vi "Calculate No of Scripts.vi"(0 "Sizes of Arrays":i32[](array[numeric]), 5 "Linked? Array":bool[](array[boolean])) -> (4 "No of scripts":i32)   [LabVIEW 2020, in "TALOS.lvlib" / "Run Utilities.lvlib" / "Scan SBlock.lvclass"]
doc: "Creates an array of parameter's values on range <From> to <To> with either step size or number of steps. It also returns a size of the array."
uses:
  Scan SBlock.lvclass
  Scan SBlock.lvclass/Scan SBlock.ctl
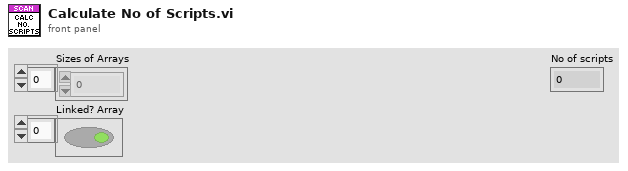
[diagram p1: front panel]
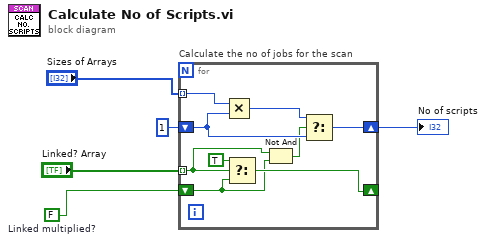
[diagram p0: block diagram]
diagram:
  w2 = FALSE  # Linked multiplied?
  n1 = for "Calculate the no of jobs for the scan" {
    tunnel: "Sizes of Arrays" -> [w14] mode=indexing
    shift-right: [w12] -> w1
    shift-left: 1 -> [w7]
    tunnel: "Linked? Array" -> [w9] mode=indexing
    shift-right: [w11] -> _
    shift-left: w2 -> [w10]
    n2 = Multiply(x=w14, y=w7) -> (x*y=w8:i32)
    n3 = Select(t=TRUE, s=w9, f=w10) -> (s? t:f=w11:bool)
    n4 = Not And(1:w10, 2:w9) -> (0:w6:bool)
    n5 = Select(t=w8, s=w6, f=w7) -> (s? t:f=w12:i32)
  }
  "No of scripts" <- w1
